vi "Set ID.vi"(8 "error in (no error)":errorcluster, 10 "ID":i32, 11 "Element Base in":refnum<class "Element Base.lvclass">) -> (0 "error out":errorcluster, 3 "Element Base out":refnum<class "Element Base.lvclass">)   [LabVIEW 2020, in "Array Example.lvlib" / "Element Base.lvclass"]
uses:
  Element Base.lvclass
  Element Base.lvclass/Element Base.ctl
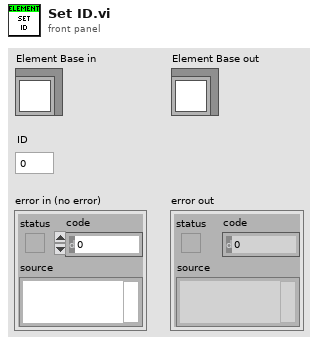
[diagram p1: front panel]
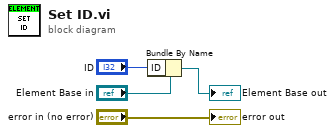
[diagram p0: block diagram]
diagram:
  n1 = Bundle By Name(cluster="Element Base in", "ID"="ID") -> (→"Element Base out":refnum<class "Element Base.lvclass">)
  "error out" <- "error in (no error)"
